vi "RngFind_ConvertSamples.vi"(0 "Input Samples":string[](array[string])) -> (14 "sensor 1":dbl, 15 "sensor 2":dbl, 16 "sensor 3":dbl, 17 "sensor 4":dbl)   [LabVIEW 2014]
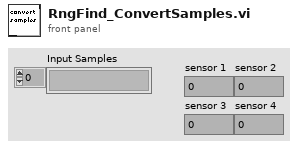
[diagram p1: front panel]
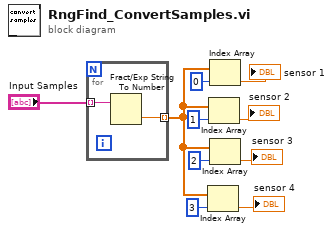
[diagram p0: block diagram]
diagram:
  n1 = for {
    tunnel: "Input Samples" -> [w12] mode=indexing
    tunnel: [w11] -> w5 mode=indexing
    n2 = Fract/Exp String To Number(string=w12) -> (number=w11:dbl)  [unwired: 3 in, 1 out]
  }
  n3 = Index Array(array=w5, index=3) -> (element=→"sensor 4":dbl)
  n4 = Index Array(array=w5, index=1) -> (element=→"sensor 2":dbl)
  n5 = Index Array(array=w5, index=0) -> (element=→"sensor 1":dbl)
  n6 = Index Array(array=w5, index=2) -> (element=→"sensor 3":dbl)
